vi "TPS_example.vi"() -> ()   [LabVIEW 2009]
panel:
  out "Array":dbl[](array[numeric])
  out "error out":errorcluster
  in  "error in (no error)":errorcluster
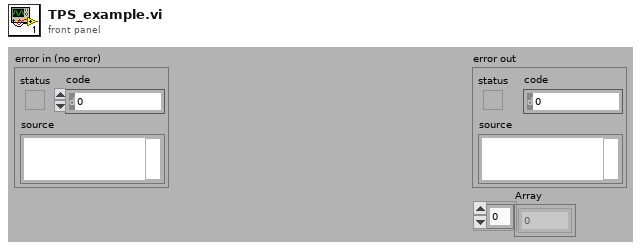
[diagram p1: front panel]
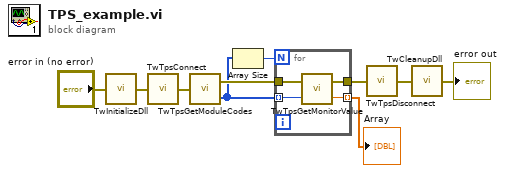
[diagram p0: block diagram]
diagram:
  n1 = call "TwInitializeDll.vi"("error in (no error)"="error in (no error)") -> ("error out"=w9:errorcluster)
  n2 = call "TwTpsConnect.vi"("error in (no error)"=w9) -> ("error out"=w8:errorcluster)
  n3 = call "TwTpsGetModuleCodes.vi"("error in (no error)"=w8) -> ("error out"=w7:errorcluster, "moduleCodeBuffer"=w2:i32[])
  n4 = Array Size(array=w2) -> (size(s)=w3:i32)
  n5 = for {
    N: w3 -> [_]
    tunnel: w7 -> [w14]
    tunnel: [w13] -> w6
    tunnel: w2 -> [w12] mode=indexing
    tunnel: [w11] -> w1 mode=indexing
    n6 = call "TwTpsGetMonitorValue.vi"("moduleCode"=w12, "error in (no error)"=w14) -> ("value"=w11:dbl, "error out"=w13:errorcluster)
  }
  "Array" <- w1
  n7 = call "TwTpsDisconnect.vi"("error in (no error)"=w6) -> ("error out"=w5:errorcluster)
  n8 = call "TwCleanupDll.vi"("error in (no error)"=w5) -> ("error out"=→"error out":errorcluster)
